vi "Write TargetName.vi"(8 "error in (no error)":errorcluster, 10 "TargetName":string, 11 "FSM.Edge in":refnum<class "FSM.Edge.lvclass">) -> (0 "error out":errorcluster, 3 "FSM.Edge out":refnum<class "FSM.Edge.lvclass">)   [LabVIEW 2020, in "FSM.Edge.lvclass"]
uses:
  FSM.Edge.lvclass
  FSM.Edge.lvclass/FSM.Edge.ctl
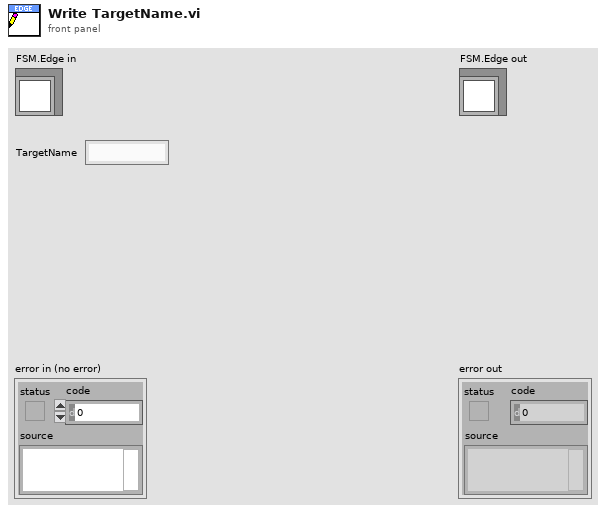
[diagram p1: front panel]
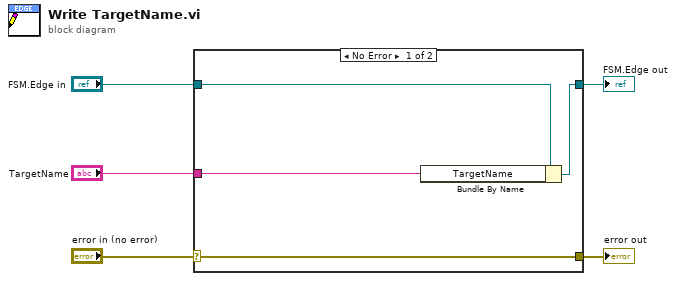
[diagram p0: block diagram]
diagram:
  n1 = case shown="No Error" "error in (no error)" {
    selector: "error in (no error)" -> [w9 w10]
    tunnel: [w9 w10] -> w4
    tunnel: [w7 w11] -> w2
    tunnel: "FSM.Edge in" -> [w8 w11]
    tunnel: "TargetName" -> [w6 _]
    frame No Error {
      n2 = Bundle By Name(cluster=w8, "TargetName"=w6) -> (w7:refnum<class "FSM.Edge.lvclass">)
    }
    frame Error {
    }
  }
  "error out" <- w4
  "FSM.Edge out" <- w2
